vi "DefaultServerDataFolder.vi"(8 "error in (no error)":errorcluster, 11 "TCP_Server_Connection_Handler in":refnum<class "TCP_Server_Connection_Handler.lvclass">) -> (0 "error out":errorcluster, 3 "TCP_Server_Connection_Handler out":refnum<class "TCP_Server_Connection_Handler.lvclass">)   [LabVIEW 2023, in "TCP_Server_Connection_Handler.lvlib" / "TCP_Server_Connection_Handler.lvclass"]
uses:
  TCP_Server_Connection_Handler.lvclass
  <vilib>/Utility/sysdir.llb/System Directory Type.ctl
  TCP_Server_Connection_Handler.lvclass/TCP_Server_Connection_Handler.ctl
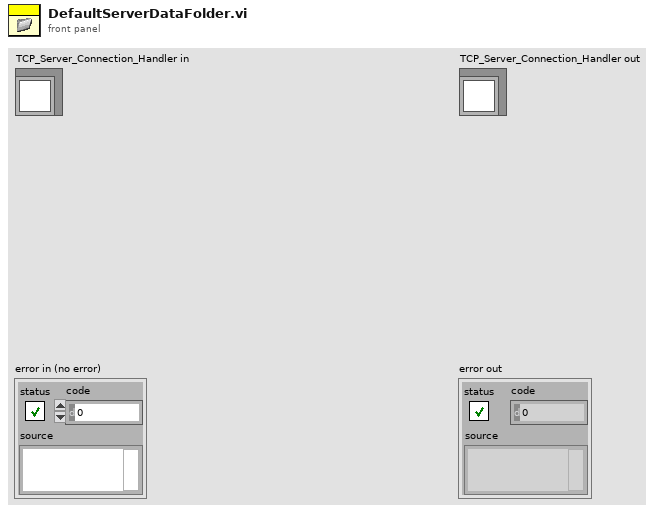
[diagram p1: front panel]
types:
  T1 = typedef "System Directory Type.ctl" = i32
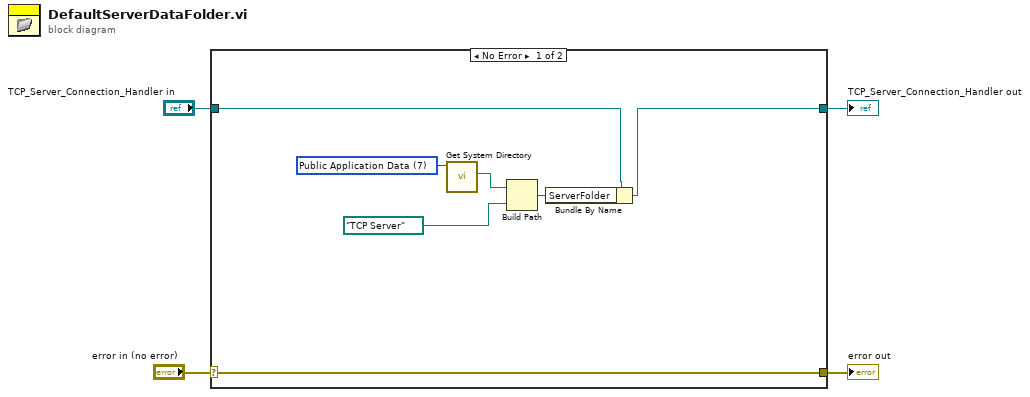
[diagram p0: block diagram]
diagram:
  n1 = case shown="No Error" "error in (no error)" {
    selector: "error in (no error)" -> [w11 w13]
    tunnel: [w11 w13] -> w3
    tunnel: [w6 w12] -> w1
    tunnel: "TCP_Server_Connection_Handler in" -> [w7 w12]
    frame No Error {
      w10 = T1 7 items=["User Home"=0, "User Desktop"=1, "User Documents"=2, "User Application Data"=3, "User Preferences"=4, "User Temporary"=5, "Public Documents"=6, "Public Application Data"=7, "Public Preferences"=8, "Public Cache"=13, "System Core Libraries"=9, "System Installed Libraries"=10, "Application Files"=11, "Boot Volume Root"=12] ("system directory type")
      n2 = call <vilib>:"Get System Directory.vi"("system directory type"=w10) -> ("system directory"=w9:path)  [unwired: 10 in]
      n3 = Build Path(base path=w9, name or relative path=path "TCP Server") -> (appended path=w5:path)
      n4 = Bundle By Name(cluster=w7, "ServerFolder"=w5) -> (w6:refnum<class "TCP_Server_Connection_Handler.lvclass">)
    }
    frame Error {
    }
  }
  "error out" <- w3
  "TCP_Server_Connection_Handler out" <- w1
